vi "sub_Acquisition Rate.vi"(1 "Divide":enum16{"120M", "60M", "30M", "15M", "7.5M"}(ring)) -> (0 "采样率":dbl)   [LabVIEW 2015]
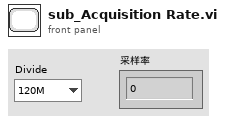
[diagram p1: front panel]
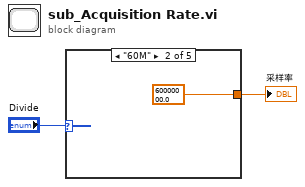
[diagram p0: block diagram]
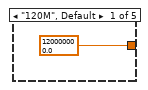
[diagram p2: hidden frame]
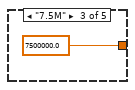
[diagram p3: hidden frame]
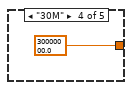
[diagram p4: hidden frame]
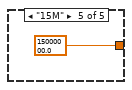
[diagram p5: hidden frame]
diagram:
  n1 = case shown="\"60M\"" "Divide" {
    tunnel: [120000000.0 ("采样率") 60000000.0 ("采样率") 7500000.0 ("采样率") 30000000.0 ("采样率") 15000000.0 ("采样率")] -> w1
    frame "120M", Default {
    }
    frame "60M" {
    }
    frame "7.5M" {
    }
    frame "30M" {
    }
    frame "15M" {
    }
  }
  "采样率" <- w1
